vi "prime_or_not.vi"() -> ()   [LabVIEW 2026]
panel:
  in  "OK Button":bool
  out "final judgement!!!":string
  in  "num":dbl
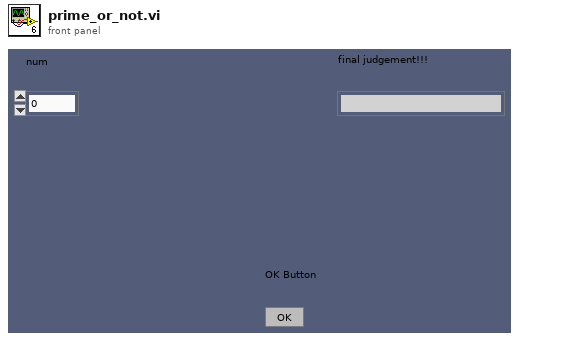
[diagram p1: front panel]
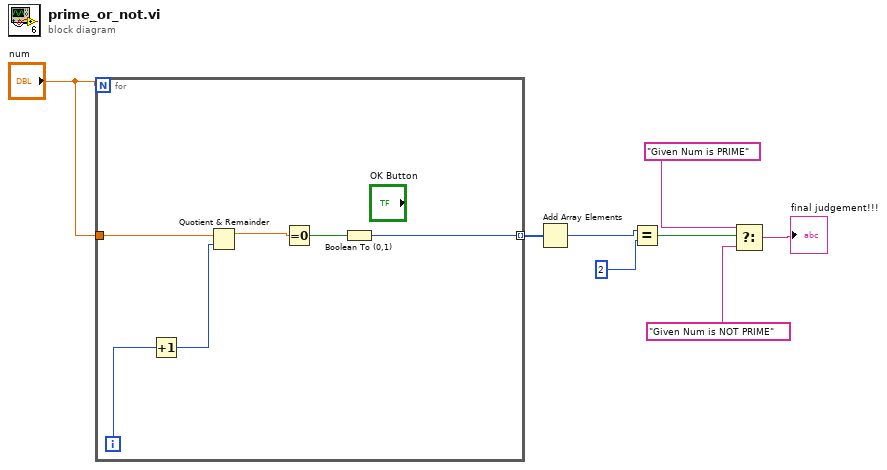
[diagram p0: block diagram]
diagram:
  n1 = for {
    N: "num" -> [_]
    tunnel: "num" -> [w14]
    tunnel: [w9] -> w7 mode=indexing
    i -> [w13]
    n2 = Increment(x=w13) -> (x+1=w12:i32)
    n3 = Quotient & Remainder(x=w14, y=w12) -> (x-y*floor(x/y)=w11:dbl)  [unwired: 1 out]
    n4 = Equal To 0?(x=w11) -> (x = 0?=w10:bool)
    n5 = Boolean To (0,1)(Boolean=w10) -> (0, 1=w9:i16)
  }
  n6 = Add Array Elements(numeric array=w7) -> (sum=w6:i16)
  n7 = Equal?(x=w6, y=2) -> (x = y?=w4:bool)
  n8 = Select(t="Given Num is PRIME", s=w4, f="Given Num is NOT PRIME") -> (s? t:f=→"final judgement!!!":string)
